vi "removeDup_valveRatios.vi"(10 "Ratios":dbl[](array[numeric]), 11 "Valves":u16[](array[numeric])) -> (2 "Ratio with Dup Removed":dbl[](array[numeric]), 3 "Valves with Dup Removed":u16[](array[numeric]))   [LabVIEW 2016]
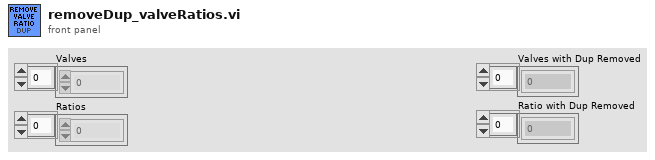
[diagram p1: front panel]
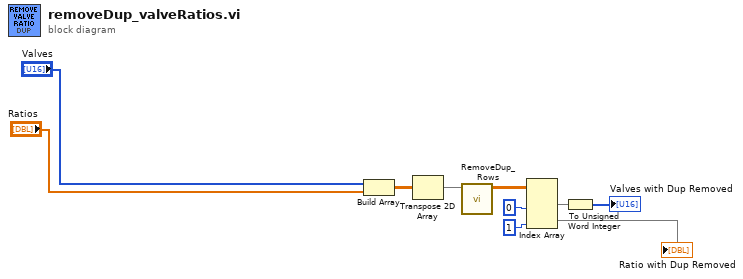
[diagram p0: block diagram]
diagram:
  n1 = Build Array("Valves", "Ratios") -> (w10:dbl[][])
  n2 = Transpose 2D Array(2D array=w10) -> (transposed array=w9:dbl[][])
  n3 = call "RemoveDup_Rows.vi"("2d Array"=w9) -> ("Array With Dup Rows Removed"=w8:dbl[][])  [unwired: 10 in]
  n4 = Index Array(array=w8, index (col) #1=0 ("disabled index (col)"), index (col) #2=1 ("index (col)")) -> (element #1=w5:dbl[], element #2=→"Ratio with Dup Removed":dbl[])  [unwired: 2 in]
  n5 = To Unsigned Word Integer(number=w5) -> (unsigned 16bit integer=→"Valves with Dup Removed":u16[])
